vi "WAM_Database_log.vi"(0 "log file path":path, 2 "results file path in":path[](array[path]), 3 "Message_In(ary)":string[](array[string])=["Overall Status:  PASS", "Serial Number: WAM-000698", "Receive Power Supply Consumption Limits : Pass", "Receiver Input Frequency : Pass", "Receiver Gain : Pass", "Receiver Noise Figure : Pass", "Transmit Output Frequency : Pass", "Transmit Power Supply Consumption Limits : Pass", "Transmit In-Band Output Peak Power : Pass", "Harmonics : Pass", "Reference Source Port Return Loss : Pass", "Transmit Power Flatness : Pass", "Temperature Sensors : Pass", "Bounce Test : Pass", "Post Process Rev: 1.0.9"], 5 "error in (no error)":errorcluster, 6 "-sid":string, 7 "Test Time":string, 8 "Ver_Tags(ary)":string[](array[string]), 9 "Enable(t)":bool=TRUE, 10 "-dbid(ary)":string[](array[string]), 11 "Run Python (t)":bool, 13 "ProcessAsError(t)":bool, 17 "Errors In":string[](array[string])) -> (14 "logfileout":path, 19 "error out":errorcluster)   [LabVIEW 2018]
uses:
  Tetra_Globals.vi
  Infrastructure/Test Parameter Globals_1.0.0.vi
  Initialize References/Sequence Globals.vi
  <vilib>/Utility/file.llb/Write Delimited Spreadsheet (string).vi
panel:
  out "size(s)":i32
  out "py Script path":path
  out "DB_Write_Success(t)":bool
  out "TestResult(ary)":string[](array[string])=["Overall Status:  PASS", "Serial Number: WAM-000698", "Receive Power Supply Consumption Limits : Pass", "Receiver Input Frequency : Pass", "Receiver Gain : Pass", "Receiver Noise Figure : Pass", "Transmit Output Frequency : Pass", "Transmit Power Supply Consumption Limits : Pass", "Transmit In-Band Output Peak Power : Pass", "Harmonics : Pass", "Reference Source Port Return Loss : Pass", "Transmit Power Flatness : Pass", "Temperature Sensors : Pass", "Bounce Test : Pass", "Post Process Rev: 1.0.9"]
  out "standard error":string
  out "standard output":string
  out "Tags(ary)":string[](array[string])
  out "computer":string
  out "tbid":string
  out "delimiter":string
  out "FileData(ary)":string[](array[string])
  out "File_Header(ary)":string[](array[string])
  in  "File Delimiter":i32(ring) items=["Comma Delimited (.csv)", "Tab Delimited (.txt)"]
  out "DataHeader":string[](array[string])=["DATE", "ssid", "attenid", "txid", "rxid", "bid"]
  out "new_file(t)":bool
  out "TestHeader":string[](array[string])=["TEST_BENCH_ID", "COMP_NAME", "ATTEN_FILE", "TX_FILE", "RX_FILE", "BOUNCE_FILE"]
  out "results file path str(ary)":string[](array[string])
  out "StatusResult(ary)":string[](array[string])
  out "StatusName(ary)":string[](array[string])
  out "date/time string":string
  out "logfilepath_full(str)":string
  # "C:\\RageATE Results\\REV-C_TETRA_TX-ATTEN\\6_9_2023\\REV-C_TETRA_TX-ATTEN_SN_WAM-000104_2232_060923-114224.csv\t\nC:\\RageATE Results\\WAM-C_BOUNCE\\6_9_2023\\WAM-C_BOUNCE_SN_WAM-000104_2232_060923-114314.csv\t\nC:\\RageATE Results\\REV-C_TETRA_TX-PROD\\6_9_2023\\REV-C_TETRA_TX-PROD_SN_WAM-000104_2232_060923-114406.csv\t\nC:\\RageATE Results\\REV-C_TETRA_RX-PROD\\6_9_2023\\REV-C_TETRA_RX-PROD_SN_WAM-000104_2232_060923-120559.csv"
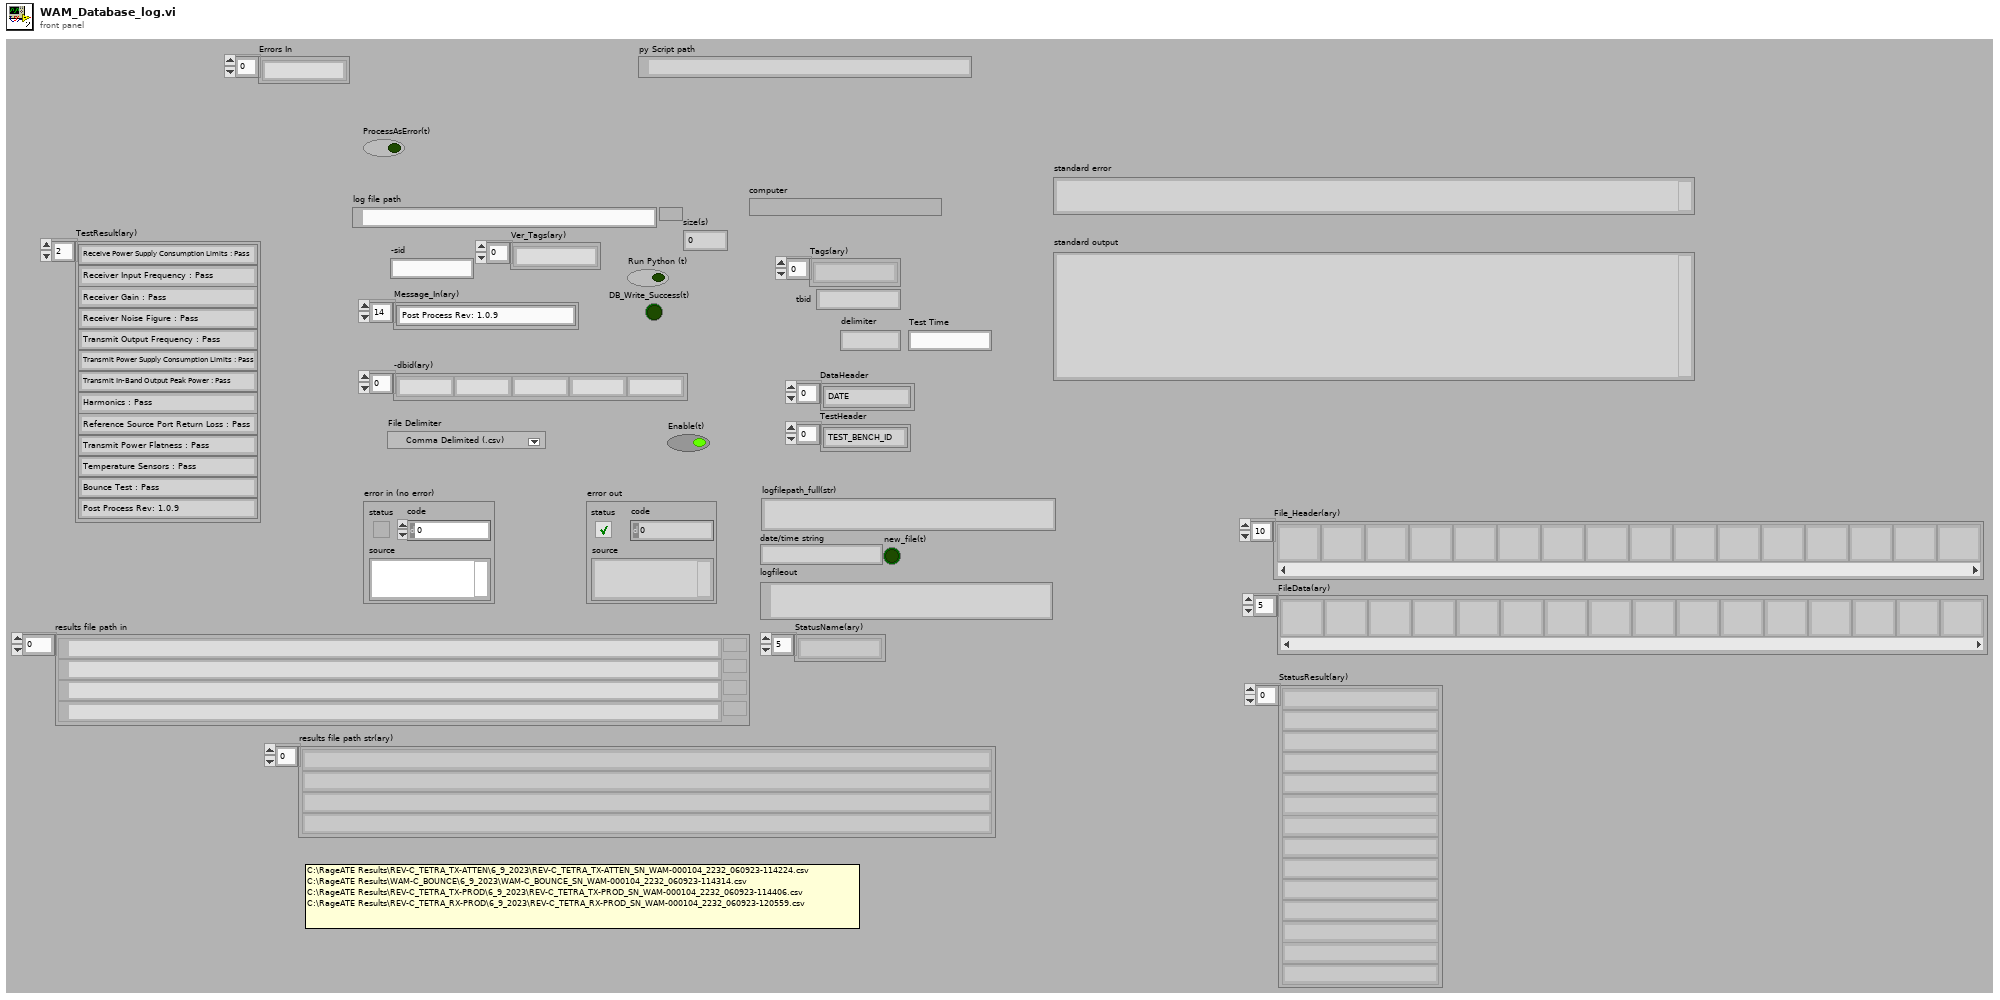
[diagram p1: front panel]
types:
  T1 = enum16{"open", "replace", "create", "open or create", "replace or create", "replace or create with confirmation"}
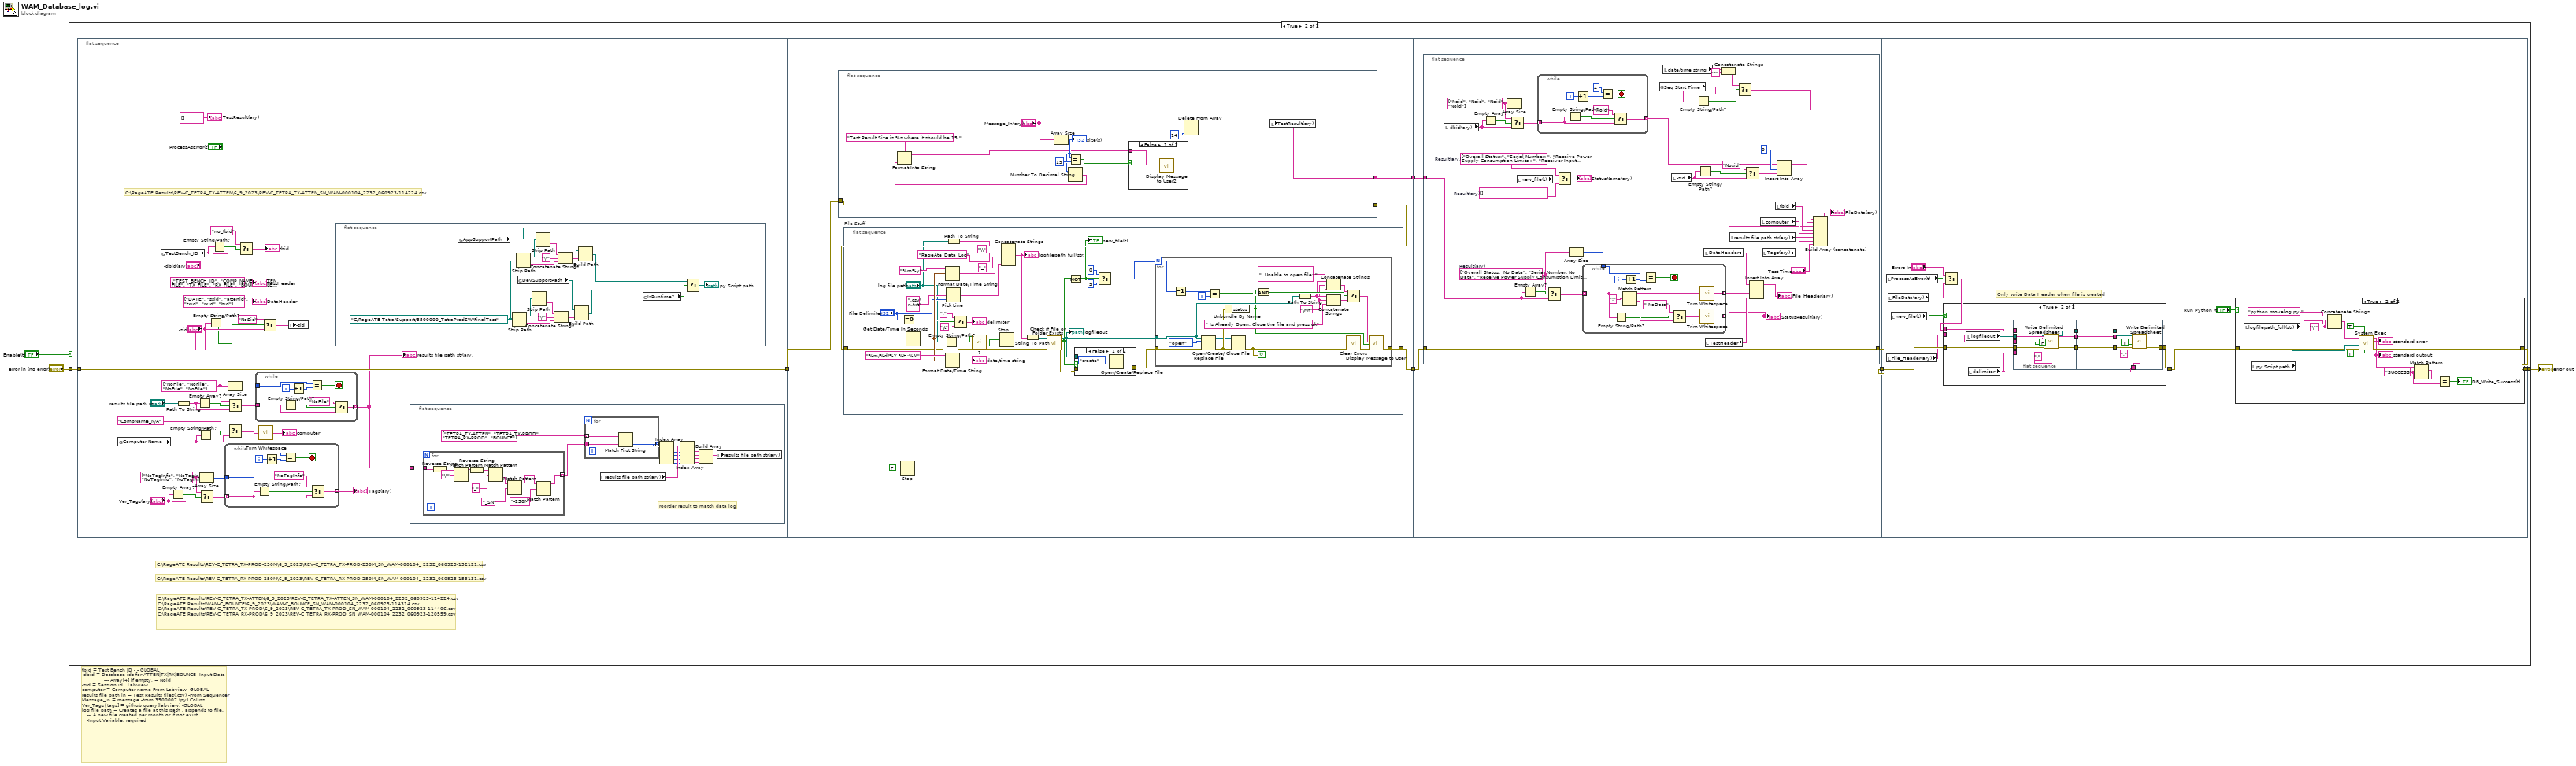
[diagram p0: block diagram]
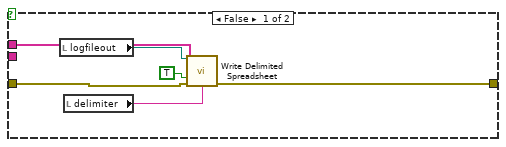
[diagram p5: hidden frame]
diagram:
  # "tbid = Test Bench ID - - GLOBAL \n-dbid = Database ids for ATTEN|TX|RX|BOUNCE -Input Data\n              --- Array[4] if empty, = Noid\n-sid = Session id , Labview\ncomputer = Computer name From Labview -GLOBAL\nresults file path in = Test Results files(.csv) -From Sequencer\nMessage_in = message -from 3500007 (py) Colins\nVer_Tags{tags] = github query(labview) -GLOBAL\nlog file path = Creates a file at this path , appends to file.\n   --- A new file created per month or if not exist\n   -Input Variable, required"
  n1 = case shown="True" "Enable(t)" {
    tunnel: [w4 w6] -> w3
    tunnel: "error in (no error)" -> [w4 w8]
    frame False {
    }
    frame True {
      # "C:\\RageATE Results\\REV-C_TETRA_TX-PROD-250M\\6_9_2023\\REV-C_TETRA_TX-PROD-250M_SN_WAM-000104_ 2232_060923-152121.csv"
      # "C:\\RageATE Results\\REV-C_TETRA_RX-PROD-250M\\6_9_2023\\REV-C_TETRA_RX-PROD-250M_SN_WAM-000104_ 2232_060923-153131.csv"
      # "C:\\RageATE Results\\REV-C_TETRA_TX-ATTEN\\6_9_2023\\REV-C_TETRA_TX-ATTEN_SN_WAM-000104_2232_060923-114224.csv\t\nC:\\RageATE Results\\WAM-C_BOUNCE\\6_9_2023\\WAM-C_BOUNCE_SN_WAM-000104_2232_060923-114314.csv\t\nC:\\RageATE Results\\REV-C_TETRA_TX-PROD\\6_9_2023\\REV-C_TETRA_TX-PROD_SN_WAM-000104_2232_060923-114406.csv\t\nC:\\RageATE Results\\REV-C_TETRA_RX-PROD\\6_9_2023\\REV-C_TETRA_RX-PROD_SN_WAM-000104_2232_060923-120559.csv"
      n2 = flat-sequence {
        tunnel: w8 -> [w27]
        tunnel: [w27] -> w11
        tunnel: [w107] -> w10
        tunnel: w11 -> [w104]
        tunnel: [w106] -> w5
        tunnel: [w177] -> w9
        tunnel: w10 -> [w178]
        tunnel: w5 -> [w176]
        tunnel: w9 -> [w243]
        tunnel: [w244] -> w7
        tunnel: w7 -> [w281]
        tunnel: [w282] -> w6
        frame #0 {
          w23 = string[] ["NoTagInfo", "NoTagInfo", "NoTagInfo", "NoTagInfo"] ("Ver_Tags(ary)")
          w25 = string[] ["NoFile", "NoFile", "NoFile", "NoFile"] ("t")
          # "C:\\RageATE Results\\REV-C_TETRA_TX-ATTEN\\6_9_2023\\REV-C_TETRA_TX-ATTEN_SN_WAM-000104_2232_060923-114224.csv"
          n3 = global read "Test Parameter Globals_1.0.0.vi" "Computer Name"() -> (w32:string)
          n4 = global read "Tetra_Globals.vi" "TestBench_ID"() -> (w34:string)
          n5 = Empty Array?(array="Ver_Tags(ary)") -> (empty?=w28:bool)
          n6 = Path To String(path="results file path in") -> (string=w38:string[])
          n7 = Empty Array?(array=w38) -> (empty?=w39:bool)
          n8 = Empty String/Path?(string/path=w32) -> (empty?=w31:bool)
          n9 = Array Size(array=w23) -> (size(s)=w22:i32)
          n10 = Select(t=w23, s=w28, f="Ver_Tags(ary)") -> (s? t:f=w29:string[])
          n11 = Empty String/Path?(string/path="-sid") -> (empty?=w17:bool)
          n12 = Empty String/Path?(string/path=w34) -> (empty?=w37:bool)
          n13 = while {
            tunnel: w29 -> [w93] mode=indexing
            tunnel: [w92] -> w30 mode=indexing
            tunnel: w22 -> [w89]
            i -> [w88]
            stop <- w90 stop-if-true
            n14 = Empty String/Path?(string/path=w93) -> (empty?=w94:bool)
            n15 = Increment(x=w88) -> (x+1=w87:i32)
            n16 = Equal?(x=w89, y=w87) -> (x = y?=w90:bool)
            n17 = Select(t="NoTagInfo", s=w94, f=w93) -> (s? t:f=w92:string)
          }
          "Tags(ary)" <- w30
          n18 = Array Size(array=w25) -> (size(s)=w24:i32)
          n19 = Select(t="CompName_N/A" ("Computer Name"), s=w31, f=w32) -> (s? t:f=w33:string)
          n20 = Select(t=w25, s=w39, f=w38) -> (s? t:f=w40:string[])
          n21 = Select(t="no_tbid", s=w37, f=w34) -> (s? t:f=→"tbid":string)
          n22 = while {
            tunnel: w40 -> [w101] mode=indexing
            tunnel: [w100] -> w12 mode=indexing
            tunnel: w24 -> [w95]
            i -> [w98]
            stop <- w96 stop-if-true
            n23 = Empty String/Path?(string/path=w101) -> (empty?=w102:bool)
            n24 = Increment(x=w98) -> (x+1=w97:i32)
            n25 = Equal?(x=w95, y=w97) -> (x = y?=w96:bool)
            n26 = Select(t="NoFile", s=w102, f=w101) -> (s? t:f=w100:string)
          }
          "results file path str(ary)" <- w12
          n27 = call <vilib>:"Trim Whitespace.vi"("string"=w33) -> ("trimmed string"=→"computer":string)  [unwired: 1 in]
          n28 = Select(t="NoSid", s=w17, f="-sid") -> (s? t:f=w19:string)
          n29 = local write "-sid"(w19) -> ()
          n30 = flat-sequence {
            frame #0 {
              w43 = path "C:/RageATE-Tetra/Support/3500000_TetraProdSW/FinalTest" ("working directory")
              n31 = global read "Sequence Globals.vi" "AppSupportPath"() -> (w44:path)
              n32 = Strip Path(path=w43) -> (stripped path=w56:path, name=w53:string)
              n33 = Strip Path(path=w43) -> (stripped path=w45:path, name=w47:string)
              n34 = global read "Sequence Globals.vi" "DevSupportPath"() -> (w55:path)
              n35 = Strip Path(path=w56) -> (name=w54:string)  [unwired: 1 out]
              n36 = Strip Path(path=w45) -> (name=w46:string)  [unwired: 1 out]
              n37 = Concatenate Strings(w54, "\\" ("string"), w53) -> (w51:string)
              n38 = Concatenate Strings(w46, "\\" ("string"), w47) -> (w49:string)
              n39 = Build Path(base path=w55, name or relative path=w51) -> (appended path=w50:path)
              n40 = Build Path(base path=w44, name or relative path=w49) -> (appended path=w42:path)
              n41 = global read "Sequence Globals.vi" "IsRuntime?"() -> (w58:bool)
              n42 = Select(t=w42, s=w58, f=w50) -> (s? t:f=→"py Script path":path)
            }
          }
          n43 = flat-sequence {
            tunnel: w12 -> [w72]
            frame #0 {
              # "roorder result to match data log"
              n44 = for {
                tunnel: w72 -> [w85] mode=indexing
                tunnel: [w76] -> w71 mode=indexing
                n45 = Reverse String(1:w85) -> (0:w84:string)
                n46 = Match Pattern(string=w84, regular expression="\\") -> (before substring=w83:string)  [unwired: 1 in, 3 out]
                n47 = Reverse String(1:w83) -> (0:w82:string)
                n48 = Match Pattern(string=w82, regular expression="_") -> (after substring=w80:string)  [unwired: 1 in, 3 out]
                n49 = Match Pattern(string=w80, regular expression="_SN") -> (before substring=w78:string)  [unwired: 1 in, 3 out]
                n50 = Match Pattern(string=w78, regular expression="-250M") -> (before substring=w76:string)  [unwired: 1 in, 3 out]
              }
              n51 = for {
                tunnel: w71 -> [w75]
                tunnel: string[] ["TETRA_TX-ATTEN", "TETRA_TX-PROD", "TETRA_RX-PROD", "BOUNCE"] ("string") -> [w74] mode=indexing
                tunnel: [w73] -> w68 mode=indexing
                n52 = Match First String(2:w75, 3:w74) -> (0:w73:i32)  [unwired: 1 out]
              }
              n53 = local read "results file path str(ary)"() -> (w69:string[])
              n54 = Index Array(array=w68) -> (element #1=w67:i32, element #2=w66:i32, element #3=w65:i32, element #4=w64:i32)  [unwired: 4 in]
              n55 = Index Array(array=w69, index #1=w67, index #2=w66, index #3=w65, index #4=w64) -> (element #1=w63:string, element #2=w62:string, element #3=w61:string, element #4=w60:string)
              n56 = Build Array(w63, w62, w61, w60) -> (w59:string[])
              n57 = local write "results file path str(ary)"(w59) -> ()
            }
          }
          "TestHeader" <- string[] ["TEST_BENCH_ID", "COMP_NAME", "ATTEN_FILE", "TX_FILE", "RX_FILE", "BOUNCE_FILE", "RageATE_Ver", "TetraLabGUI_Ver", "3500004_Ver", "3500007_Ver", "Elapsed Time"] ("new element/subarray")
          "DataHeader" <- string[] ["DATE", "ssid", "attenid", "txid", "rxid", "bid"]
          "TestResult(ary)" <- string[] [] ("TestResult(ary)")
        }
        frame #1 {
          n58 = flat-sequence {
            tunnel: [w116] -> w106
            tunnel: w104 -> [w115]
            tunnel: [w115] -> w103
            frame #0 {
              n59 = Array Size(array="Message_In(ary)") -> (size(s)=w110:i32)
              "size(s)" <- w110
              n60 = Number To Decimal String(number=w110) -> (decimal integer string=w109:string)  [unwired: 1 in]
              n61 = Format Into String(format string="Test Result Size is %s where it should be 15 ", w109) -> (resulting string=w108:string)  [unwired: 2 in, 1 out]
              n62 = Equal?(x=w110, y=15) -> (x = y?=w112:bool)
              n63 = case shown="False" w112 {
                tunnel: w108 -> [w118 _]
                frame False {
                  n64 = call "Display Message to User2"("Message"=w118) -> ()  [unwired: 9 in, 2 out]
                }
                frame True {
                }
              }
              n65 = Delete From Array(array="Message_In(ary)", index=14) -> (array with subset deleted=w116:string[])  [unwired: 1 in, 1 out]
              n66 = local write "TestResult(ary)"(w116) -> ()
            }
          }
          n67 = flat-sequence "File Stuff" {
            tunnel: [w129] -> w107
            tunnel: w103 -> [w123]
            frame #0 {
              n68 = Equal To 0?(x="File Delimiter") -> (x = 0?=w137:bool)
              n69 = Get Date/Time In Seconds() -> (seconds since 1Jan1904=w140:timestamp)
              n70 = Empty String/Path?(string/path="log file path") -> (empty?=w131:bool)
              n71 = Format Date/Time String(time format string (%c)="%m%y" ("format string"), seconds (now)=w140) -> (date/time string=w147:string)  [unwired: 1 in]
              n72 = Format Date/Time String(time format string (%c)="%m/%d/%Y %H:%M" ("format string"), seconds (now)=w140) -> (date/time string=→"date/time string":string)  [unwired: 1 in]
              n73 = Pick Line(multi-line string=".csv\n.txt", line index="File Delimiter") -> (output string=w138:string)  [unwired: 1 in]
              n74 = Path To String(path="log file path") -> (string=w148:string)
              n75 = Select(t=",", s=w137, f="\t") -> (s? t:f=→"delimiter":string)
              n76 = call "?"("Enable"=w131, "error in (no error)"=w123) -> ("OK"=w130:bool, "error out"=w128:errorcluster)  [unwired: 16 in]
              n77 = Stop(stop? (T)=w130) -> ()
              n78 = Concatenate Strings(w148, "\\" ("string"), "RageAte_Data_Log" ("string"), "_" ("string"), w147, w138) -> (w146:string)
              "logfilepath_full(str)" <- w146
              n79 = String To Path(string=w146) -> (path=w149:path)
              n80 = call <vilib>:"Check if File or Folder Exists.vi"("error in (no error)"=w128, "path"=w149) -> ("error out"=w119:errorcluster, "file or folder exists?"=w121:bool, "dup path"=w122:path)  [unwired: 7 in]
              "logfileout" <- w122
              n81 = Not(x=w121) -> (.not. x?=w124:bool)
              "new_file(t)" <- w124
              n82 = case shown="False" w121 {
                tunnel: w122 -> [w153 _]
                tunnel: [w151 w154] -> w120
                tunnel: w119 -> [_ w154]
                frame False {
                  n83 = Open/Create/Replace File(file path (use dialog)=w153, operation (0:open)=T1."create") -> (error out=w151:errorcluster)  [unwired: 4 in, 2 out]
                }
                frame True {
                }
              }
              n84 = Select(t=0, s=w124, f=5) -> (s? t:f=w125:i32)
              n85 = for {
                N: w125 -> [w159]
                tunnel: w120 -> [w175]
                tunnel: w122 -> [w173]
                tunnel: [w171] -> w129
                i -> [w160]
                stop <- w168 continue-if-true
                w155 = "\r\n"
                n86 = Decrement(x=w159) -> (x-1=w158:i32)
                n87 = Open/Create/Replace File(file path (use dialog)=w173, error in=w175, operation (0:open)=T1."open") -> (refnum out=w169:refnum<file>, error out=w170:errorcluster)  [unwired: 3 in, 1 out]
                n88 = Equal?(x=w158, y=w160) -> (x = y?=w167:bool)
                n89 = Unbundle By Name(w170) -> ("status"=w166:bool)
                n90 = Close File(refnum=w169, error in=w170) -> (error out=w168:errorcluster)  [unwired: 1 out]
                n91 = And(x=w166, y=w167) -> (x .and. y?=w164:bool)
                n92 = Path To String(path=w173) -> (string=w163:string)
                n93 = Concatenate Strings(w163, w155, "  Unable to open file: " ("t")) -> (w162:string)
                n94 = Concatenate Strings(w163, w155, " Is Already Open. Close the file and press ok" ("string")) -> (w165:string)
                n95 = Select(t=w162, s=w164, f=w165) -> (s? t:f=w161:string)
                n96 = call <vilib>:"Clear Errors.vi"("error in (no error)"=w168) -> ("error out"=w172:errorcluster)  [unwired: 5 in, 1 out]
                n97 = call "Display Message to User"("error in (no error)"=w172, "Enable"=w166, "Message"=w161) -> ("error out"=w171:errorcluster)  [unwired: 7 in, 1 out]
              }
            }
          }
          n98 = Stop(stop? (T)=FALSE) -> ()
        }
        frame #2 {
          n99 = flat-sequence {
            tunnel: w178 -> [w194]
            tunnel: [w194] -> w177
            tunnel: w176 -> [w189]
            frame #0 {
              w190 = string[] ["Overall Status:  No Data", "Serial Number: No Data", "Receive Power Supply Consumption Limits : No Data", "Receiver Input Frequency : No Data", "Receiver Gain : No Data", "Receiver Noise Figure : No Data", "Transmit Output Frequency : No Data", "Transmit Power Supply Consumption Limits : No Data", "Transmit In-Band Output Peak Power : No Data", "Harmonics : No Data", "Reference Source Port Return Loss : No Data", "Transmit Power Flatness : No Data", "Temperature Sensors : No Data", "Bounce Test : No Data"]  # Result(ary)
              w195 = string[] []  # Result(ary)
              w197 = string[] ["Overall Status:", "Serial Number: ", "Receive Power Supply Consumption Limits : ", "Receiver Input Frequency : ", "Receiver Gain : ", "Receiver Noise Figure : ", "Transmit Output Frequency : ", "Transmit Power Supply Consumption Limits : ", "Transmit In-Band Output Peak Power : ", "Harmonics : ", "Reference Source Port Return Loss : ", "Transmit Power Flatness : ", "Temperature Sensors : ", "Bounce Test : ", "Post Process Rev: "]  # Result(ary)
              w199 = string[] ["Noid", "Noid", "Noid", "Noid"] ("t")
              n100 = local read "-dbid(ary)"() -> (w201:string[])
              n101 = Empty Array?(array=w201) -> (empty?=w206:bool)
              n102 = Array Size(array=w199) -> ()  [unwired: 1 out]
              n103 = Select(t=w199, s=w206, f=w201) -> (s? t:f=w207:string[])
              n104 = local read "new_file(t)"() -> (w196:bool)
              n105 = Empty Array?(array=w189) -> (empty?=w191:bool)
              n106 = while {
                tunnel: w207 -> [w236] mode=indexing
                tunnel: [w235] -> w208 mode=indexing
                i -> [w232]
                stop <- w231 stop-if-true
                n107 = Empty String/Path?(string/path=w236) -> (empty?=w237:bool)
                n108 = Increment(x=w232) -> (x+1=w230:i32)
                n109 = Equal?(x=4, y=w230) -> (x = y?=w231:bool)
                n110 = Select(t="Noid", s=w237, f=w236) -> (s? t:f=w235:string)
              }
              n111 = Select(t=w190, s=w191, f=w189) -> (s? t:f=w192:string[])
              n112 = Select(t=w197, s=w196, f=w195) -> (s? t:f=→"StatusName(ary)":string[])
              n113 = Array Size(array=w190) -> (size(s)=w193:i32)
              n114 = while {
                tunnel: w192 -> [w224] mode=indexing
                tunnel: [w227] -> w210 mode=indexing
                tunnel: [w226] -> w188 mode=indexing
                tunnel: w193 -> [w222]
                i -> [w225]
                stop <- w217 stop-if-true
                n115 = Empty String/Path?(string/path=w224) -> (empty?=w218:bool)
                n116 = Match Pattern(string=w224, regular expression=":") -> (before substring=w228:string, after substring=w220:string)  [unwired: 1 in, 2 out]
                n117 = Increment(x=w225) -> (x+1=w223:i32)
                n118 = Equal?(x=w222, y=w223) -> (x = y?=w217:bool)
                n119 = Select(t=" NoData", s=w218, f=w220) -> (s? t:f=w221:string)
                n120 = call <vilib>:"Trim Whitespace.vi"("string"=w228) -> ("trimmed string"=w227:string)  [unwired: 1 in]
                n121 = call <vilib>:"Trim Whitespace.vi"("string"=w221) -> ("trimmed string"=w226:string)  [unwired: 1 in]
              }
              "StatusResult(ary)" <- w188
              n122 = global read "Test Parameter Globals_1.0.0.vi" "Seq Start Time"() -> (w185:string)
              n123 = local read "date/time string"() -> (w182:string)
              n124 = local read "-sid"() -> (w200:string)
              n125 = Empty String/Path?(string/path=w185) -> (empty?=w186:bool)
              n126 = Empty String/Path?(string/path=w200) -> (empty?=w205:bool)
              n127 = local read "DataHeader"() -> (w202:string[])
              n128 = local read "TestHeader"() -> (w209:string[])
              n129 = Concatenate Strings(w182, "*" ("string")) -> (w183:string)
              n130 = local read "results file path str(ary)"() -> (w215:string[])
              n131 = Select(t=w183, s=w186, f=w185) -> (s? t:f=w184:string)
              n132 = Select(t="Nosid", s=w205, f=w200) -> (s? t:f=w204:string)
              n133 = Insert Into Array(array=w202, new element #1=w210, new element #2=w209) -> (→"File_Header(ary)":string[])  [unwired: 1 in]
              n134 = local read "computer"() -> (w212:string)
              n135 = local read "Tags(ary)"() -> (w213:string[])
              n136 = local read "tbid"() -> (w214:string)
              n137 = Insert Into Array(array=w208, index=0, new element=w204) -> (w216:string[])
              n138 = Build Array (concatenate)(w184, w216, w188, w214, w212, w215, w213, "Test Time") -> (→"FileData(ary)":string[])
            }
          }
        }
        frame #3 {
          # "Only write Data Header when file is created"
          n139 = local read "ProcessAsError(t)"() -> (w239:bool)
          n140 = local read "File_Header(ary)"() -> (w242:string[])
          n141 = local read "FileData(ary)"() -> (w241:string[])
          n142 = local read "new_file(t)"() -> (w245:bool)
          n143 = Select(t="Errors In", s=w239, f=w241) -> (s? t:f=w240:string[])
          n144 = case shown="True" w245 {
            tunnel: w240 -> [w250 w261]
            tunnel: w242 -> [_ w258]
            tunnel: [w247 w256] -> w244
            tunnel: w243 -> [w248 w253]
            frame False {
              n145 = local read "logfileout"() -> (w246:path)
              n146 = local read "delimiter"() -> (w249:string)
              n147 = call-poly <vilib>:"Write Delimited Spreadsheet.vi"("file path (dialog if empty)"=w246, "1D data"=w250, "append to file? (new file:F)"=TRUE, "error in (no error)"=w248, "delimiter (\\t)"=w249) -> ("error out"=w247:errorcluster)  [unwired: 9 in, 1 out]
            }
            frame True {
              n148 = local read "logfileout"() -> (w252:path)
              n149 = local read "delimiter"() -> (w257:string)
              n150 = flat-sequence {
                tunnel: [w270] -> w262
                tunnel: w261 -> [w270]
                tunnel: [w269] -> w259
                tunnel: w258 -> [w268]
                tunnel: w257 -> [w267]
                tunnel: [w266] -> w255
                tunnel: w253 -> [w265]
                tunnel: w252 -> [w264]
                tunnel: [w274] -> w263
                tunnel: w262 -> [w274]
                tunnel: [w273] -> w260
                tunnel: w259 -> [w273]
                tunnel: w255 -> [w272]
                tunnel: [w272] -> w254
                tunnel: w263 -> [w278]
                tunnel: w260 -> [w280]
                tunnel: w257 -> [w277]
                tunnel: [w276] -> w256
                tunnel: w254 -> [w275]
                frame #0 {
                  (unwired) "," ("delimiter (\\t)")
                  n151 = call-poly <vilib>:"Write Delimited Spreadsheet.vi"("file path (dialog if empty)"=w264, "1D data"=w268, "append to file? (new file:F)"=FALSE, "error in (no error)"=w265, "delimiter (\\t)"=w267) -> ("new file path (Not A Path if cancelled)"=w269:path, "error out"=w266:errorcluster)  [unwired: 9 in]
                }
                frame #1 {
                }
                frame #2 {
                  (unwired) "," ("delimiter (\\t)")
                  n152 = call-poly <vilib>:"Write Delimited Spreadsheet.vi"("file path (dialog if empty)"=w280, "1D data"=w278, "append to file? (new file:F)"=TRUE, "error in (no error)"=w275, "delimiter (\\t)"=w277) -> ("error out"=w276:errorcluster)  [unwired: 9 in, 1 out]
                }
              }
            }
          }
        }
        frame #4 {
          n153 = case shown="True" "Run Python (t)" {
            tunnel: w281 -> [w284 w285]
            tunnel: [w284 w296] -> w282
            frame False {
            }
            frame True {
              w288 = "SUCCESS" ("regular expression")
              w293 = "\"" ("string")
              n154 = local read "logfilepath_full(str)"() -> (w292:string)
              n155 = local read "py Script path"() -> (w286:path)
              n156 = Concatenate Strings("python movelog.py " ("command line"), w293, w292, w293) -> (w294:string)
              n157 = call <vilib>:"System Exec.vi"("run minimized? (F)"=TRUE, "wait until completion? (T)"=TRUE, "error in (no error)"=w285, "working directory"=w286, "command line"=w294) -> ("error out"=w296:errorcluster, "standard error"=→"standard error":string, "standard output"=w290:string)  [unwired: 3 in, 1 out]
              "standard output" <- w290
              n158 = Match Pattern(string=w290, regular expression=w288) -> (match substring=w289:string)  [unwired: 1 in, 3 out]
              n159 = Equal?(x=w289, y=w288) -> (x = y?=→"DB_Write_Success(t)":bool)
            }
          }
        }
      }
    }
  }
  "error out" <- w3
